vi "waaca_file.vi"(8 "Boolean":bool, 11 "INPUT R.AVG":dbl) -> ()   [LabVIEW 2016]
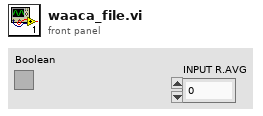
[diagram p1: front panel]
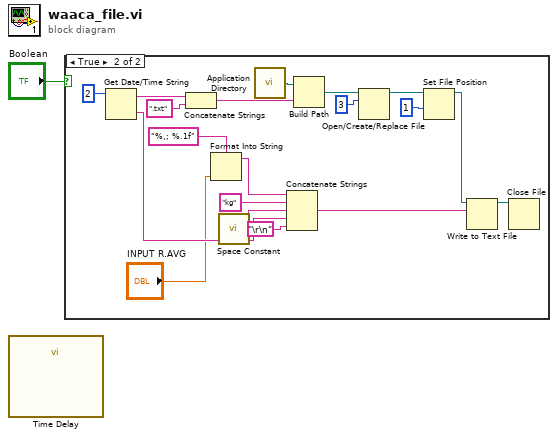
[diagram p0: block diagram]
diagram:
  n1 = call "Time Delay"() -> ()  [unwired: 11 in, 1 out]
  n2 = case shown="True" "Boolean" {
    frame False {
    }
    frame True {
      n3 = Get Date/Time String(date format (0)=2) -> (date string=w3:string, time string=w12:string)  [unwired: 2 in]
      n4 = Concatenate Strings(w3, ".txt") -> (w2:string)
      n5 = Format Into String(format string="%,; %.1f", "INPUT R.AVG") -> (resulting string=w6:string)  [unwired: 2 in, 1 out]
      n6 = call <vilib>:"Space Constant.vi"() -> ("String"=w13:string)
      n7 = call <vilib>:"Application Directory.vi"() -> ("Application Directory"=w17:path)
      n8 = Concatenate Strings(w6, "kg", w13, w12, "\r\n") -> (w18:string)
      n9 = Build Path(base path=w17, name or relative path=w2) -> (appended path=w16:path)
      n10 = Open/Create/Replace File(file path (use dialog)=w16, operation (0:open)=3) -> (refnum out=w11:refnum<file>)  [unwired: 4 in, 2 out]
      n11 = Set File Position(refnum=w11, from (0:start)=1) -> (refnum out=w10:refnum<file>)  [unwired: 2 in, 1 out]
      n12 = Write to Text File(file (use dialog)=w10, text=w18) -> (refnum out=w20:refnum<file>)  [unwired: 2 in, 2 out]
      n13 = Close File(refnum=w20) -> ()  [unwired: 1 in, 2 out]
    }
  }
